vi "Broadcast Response.vi"(8 "error in (no error)":errorcluster, 9 "Acquired Result.lvclass":refnum<class "Acquired Result.lvclass">, 10 "Topic":string, 11 "Measure Object in":refnum<class "Line Detector.lvclass">) -> (0 "error out":errorcluster, 3 "Measure Object out":refnum<class "Line Detector.lvclass">)   [LabVIEW 2016, in "Line Detector.lvclass"]
uses:
  Line Detector.lvclass
  Results/Acquired Result/Acquired Result.lvclass
  Line Detector.lvclass/Line Detector.ctl
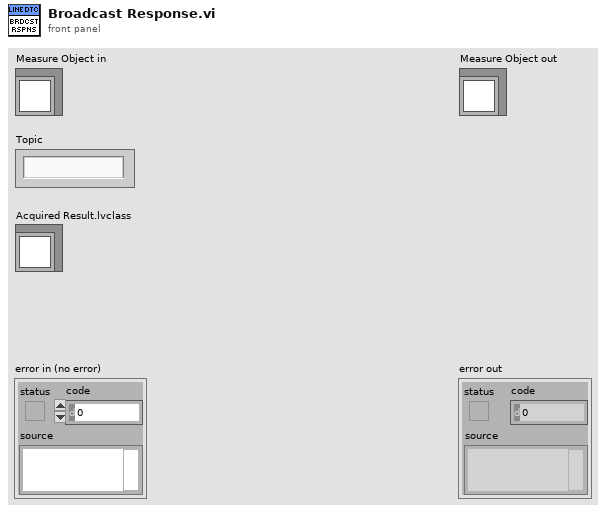
[diagram p1: front panel]
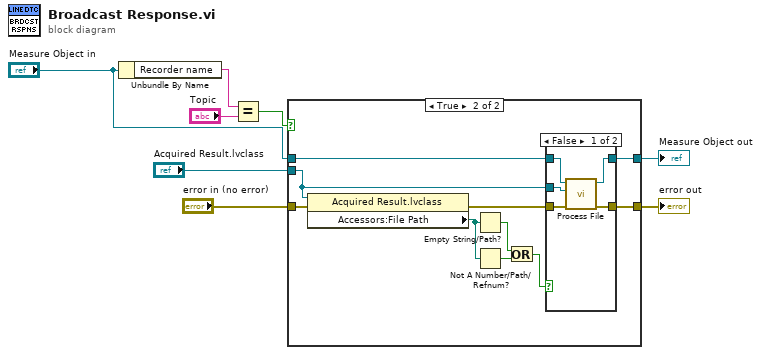
[diagram p0: block diagram]
diagram:
  n1 = Unbundle By Name("Measure Object in") -> ("Recorder name"=w8:string)
  n2 = Equal?(x=w8, y="Topic") -> (x = y?=w3:bool)
  n3 = case shown="True" w3 {
    tunnel: "Acquired Result.lvclass" -> [_ w11]
    tunnel: "error in (no error)" -> [w10 w20]
    tunnel: "Measure Object in" -> [w9 w19]
    tunnel: [w9 w17] -> w2
    tunnel: [w10 w16] -> w1
    frame False {
    }
    frame True {
      n4 = property class="Acquired Result.lvclass"(reference=w11, error in=w20) -> (error out=w18:errorcluster, "Accessors:File Path"=w15:path)  [unwired: 1 out]
      n5 = Empty String/Path?(string/path=w15) -> (empty?=w14:bool)
      n6 = Not A Number/Path/Refnum?(number/path/refnum=w15) -> (NaN/Path/Refnum?=w13:bool)
      n7 = Or(x=w14, y=w13) -> (x .or. y?=w12:bool)
      n8 = case shown="False" w12 {
        tunnel: w19 -> [w25 w27]
        tunnel: w18 -> [w24 w26]
        tunnel: [w23 w27] -> w17
        tunnel: [w22 w26] -> w16
        tunnel: w11 -> [w21 _]
        frame False {
          n9 = call-dynamic "Process File.vi"("error in (no error)"=w24, "File"=w21, "Line Detector in"=w25) -> ("error out"=w22:errorcluster, "Line Detector out"=w23:refnum<class "Line Detector.lvclass">)  [unwired: 6 in, 1 out]
        }
        frame True {
        }
      }
    }
  }
  "error out" <- w1
  "Measure Object out" <- w2
